vi "Euler_ang_Sim2Table_conv_v2(SubVI).vi"(11 "Euler Angles SIM[rad]":dbl[](array[numeric])) -> (3 "Euler Angles Table [deg]":dbl[](array[numeric]))   [LabVIEW 2017]
uses:
  <vilib>/Analysis/coordinate.llb/Euler Rotation Order.ctl
  <vilib>/Analysis/NI_AALPro.lvlib
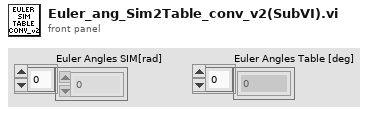
[diagram p1: front panel]
types:
  T1 = typedef "NI_AALPro.lvlib/Euler Rotation Order.ctl" = u16
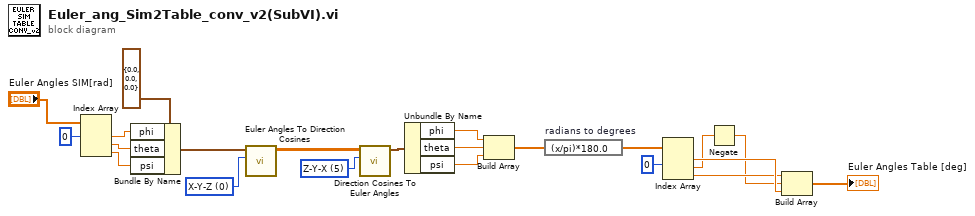
[diagram p0: block diagram]
diagram:
  w6 = T1 5 items=["X-Y-Z", "X-Z-Y", "Y-X-Z", "Y-Z-X", "Z-X-Y", "Z-Y-X", "X-Y-X", "X-Z-X", "Y-X-Y", "Y-Z-Y", "Z-X-Z", "Z-Y-Z"] ("rotation order")
  w4 = T1 0 items=["X-Y-Z", "X-Z-Y", "Y-X-Z", "Y-Z-X", "Z-X-Y", "Z-Y-X", "X-Y-X", "X-Z-X", "Y-X-Y", "Y-Z-Y", "Z-X-Z", "Z-Y-Z"] ("rotation order")
  n1 = Index Array(array="Euler Angles SIM[rad]", index #1=0 ("index")) -> (element #1=w10:dbl, element #2=w11:dbl, element #3=w12:dbl)  [unwired: 2 in]
  n2 = Bundle By Name(cluster=cluster{"phi":dbl, "theta":dbl, "psi":dbl} {"phi"=0.0, "theta"=0.0, "psi"=0.0} ("Euler Angles"), "phi"=w10, "theta"=w11, "psi"=w12) -> (w8:cluster{"phi":dbl, "theta":dbl, "psi":dbl})
  n3 = call <vilib>:"Euler Angles To Direction Cosines.vi"("rotation order"=w4, "Euler Angles"=w8) -> ("Direction Cosines"=w5:dbl[][])  [unwired: 8 in, 1 out]
  n4 = call <vilib>:"Direction Cosines To Euler Angles.vi"("rotation order"=w6, "Direction Cosines"=w5) -> ("Euler Angles"=w13:cluster{"phi":dbl, "theta":dbl, "psi":dbl})  [unwired: 8 in, 1 out]
  n5 = Unbundle By Name(w13) -> ("phi"=w15:dbl, "theta"=w14:dbl, "psi"=w16:dbl)
  n6 = Build Array(w15, w14, w16) -> (w17:dbl[])
  n7 = expression code="(x/pi)*180.0" "radians to degrees"(w17) -> (w18:dbl[])
  n8 = Index Array(array=w18, index #1=0 ("index")) -> (element #1=w20:dbl, element #2=w1:dbl, element #3=w3:dbl)  [unwired: 2 in]
  n9 = Negate(x=w1) -> (-x=w2:dbl)
  n10 = Build Array(w3, w2, w20) -> (→"Euler Angles Table [deg]":dbl[])
